vi "init.vi"(8 "error in (no error)":errorcluster, 10 "Variant":variant, 11 "NI-9237 in":refnum<class "NI-9237.lvclass">) -> (0 "error out":errorcluster, 3 "NI-9237 out":refnum<class "NI-9237.lvclass">)   [LabVIEW 2025, in "Wheatstone Bridge.lvlib" / "NI-9237.lvclass"]
uses:
  NI-9237.lvclass
  NI-9237.lvclass/NI-9237.ctl
  Wheatstone Bridge/Wheatstone Bridge.lvclass
  <resource>/objmgr/daqmx.rc
  <vilib>/DAQmx/create/channels.llb/DAQmx Create Channel (AI-Torque-Bridge-Two-Point-Linear).vi
  <vilib>/DAQmx/configure/timing.llb/DAQmx Timing (Sample Clock).vi
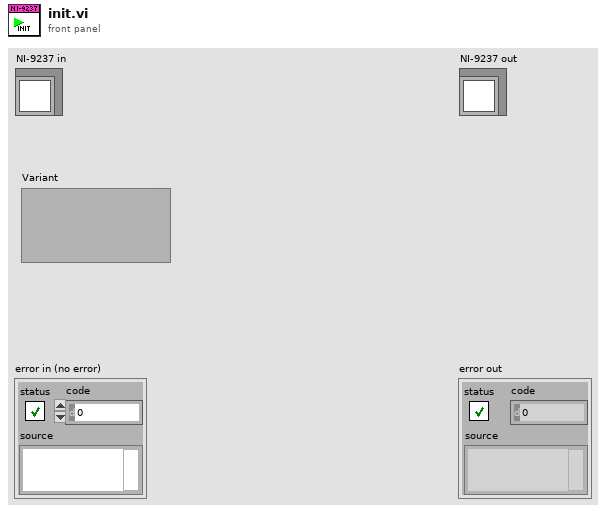
[diagram p1: front panel]
types:
  T1 = cluster{"bridge configuration":i32, "voltage excitation source":i32, "voltage excitation value":dbl, "nominal bridge resistance":dbl}
  T2 = cluster{"first electrical value":dbl, "second electrical value":dbl, "electrical units":i32, "first physical value":dbl, "second physical value":dbl, "physical units":i32}
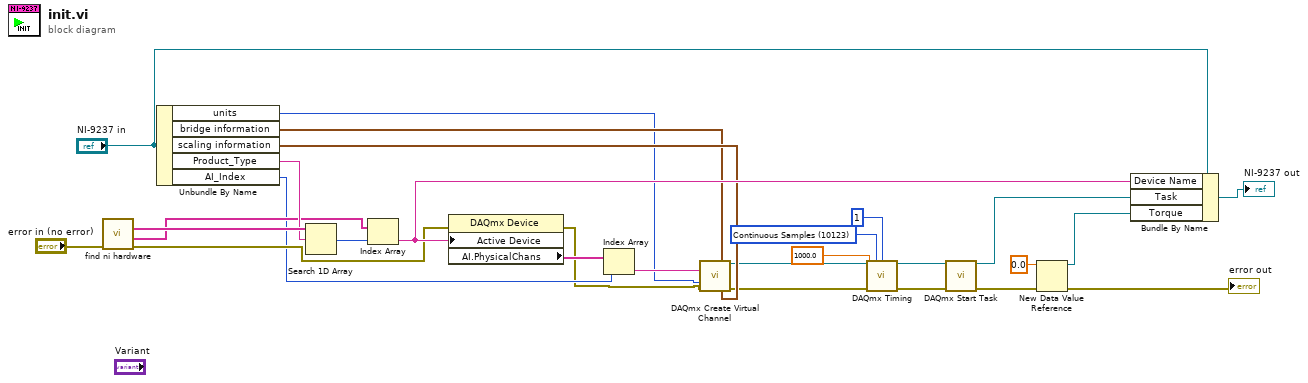
[diagram p0: block diagram]
diagram:
  w10 = 10123 items=["Finite Samples"=10178, "Continuous Samples"=10123, "Hardware Timed Single Point"=12522] ("sample mode")
  n1 = call "find ni hardware.vi"("error in (no error)"="error in (no error)") -> ("error out"=w21:errorcluster, "DevNames"=w24:tag[], "ProductType"=w28:string[])  [unwired: 7 in, 1 out]
  n2 = Unbundle By Name("NI-9237 in") -> ("units"=w13:i32, "bridge information"=w14:T1, "scaling information"=w15:T2, "Product_Type"=w27:string, "AI_Index"=w19:u16)
  n3 = Search 1D Array(1D array=w28, element=w27) -> (index of element=w23:i32)  [unwired: 1 in]
  n4 = Index Array(array=w24, index=w23) -> (element=w22:tag)
  n5 = property class="DAQmx Device"(error in=w21, "Active Device"=w22) -> (error out=w16:errorcluster, "AI.PhysicalChans"=w18:tag[])  [unwired: 1 in, 1 out]
  n6 = Index Array(array=w18, index=w19) -> (element=w17:tag)
  n7 = call-poly <vilib>:"DAQmx Create Virtual Channel.vi"("bridge information"=w14, "physical channels"=w17, "units"=w13, "error in"=w16, "scaling information"=w15) -> ("task out"=w11:refnum<k21>, "error out"=w12:errorcluster)  [unwired: 9 in]
  n8 = call-poly <vilib>:"DAQmx Timing.vi"("task/channels in"=w11, "sample mode"=w10, "samples per channel"=1, "rate"=1000.0, "error in"=w12) -> ("task out"=w7:refnum<k21>, "error out"=w6:errorcluster)  [unwired: 9 in]
  n9 = call <vilib>:"DAQmx Start Task.vi"("task/channels in"=w7, "error in"=w6) -> ("task out"=w5:refnum<k21>, "error out"=w3:errorcluster)  [unwired: 12 in]
  n10 = New Data Value Reference(data value=0.0, error in=w3) -> (data value reference=w1:refnum<data-value>, error out=→"error out":errorcluster)
  n11 = Bundle By Name(cluster="NI-9237 in", "Device Name"=w22, "Task"=w5, "Torque"=w1) -> (→"NI-9237 out":refnum<class "NI-9237.lvclass">)
